vi "Read Log Root.vi"(8 "error in (no error)":errorcluster, 11 "File Logger in":refnum<class "File Logger.lvclass">) -> (0 "error out":errorcluster, 2 "Log Root":path, 3 "File Logger out":refnum<class "File Logger.lvclass">)   [LabVIEW 2020, in "Logging.lvlib" / "File Logger.lvclass"]
uses:
  File Logger.lvclass
  File Logger.lvclass/File Logger.ctl
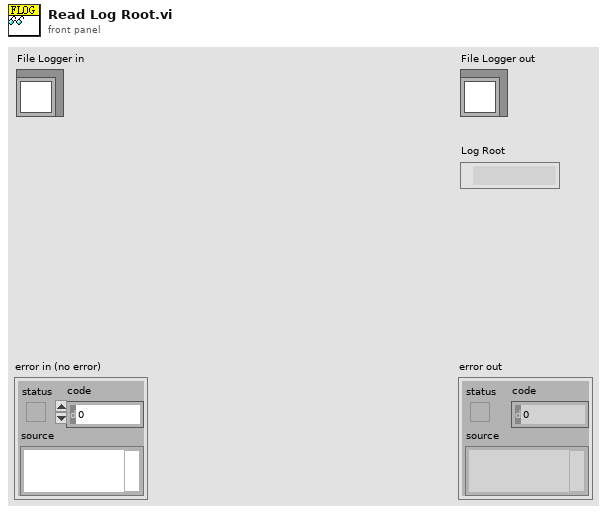
[diagram p1: front panel]
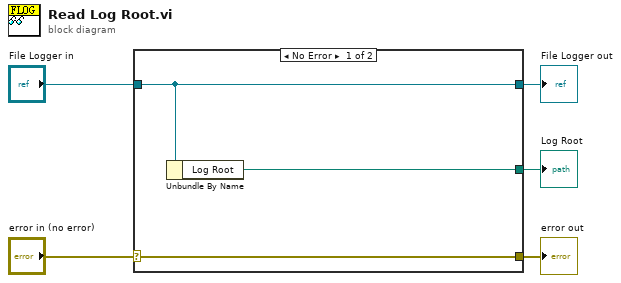
[diagram p0: block diagram]
diagram:
  n1 = case shown="No Error" "error in (no error)" {
    selector: "error in (no error)" -> [w8 w9]
    tunnel: [w8 w9] -> w4
    tunnel: [w7 w10] -> w2
    tunnel: "File Logger in" -> [w7 w10]
    tunnel: [w6 _] -> w1
    frame No Error {
      n2 = Unbundle By Name(w7) -> ("Log Root"=w6:path)
    }
    frame Error {
    }
  }
  "error out" <- w4
  "File Logger out" <- w2
  "Log Root" <- w1
